vi "VG_Array_OCVCELL.vi"() -> ()   [LabVIEW 2020]
panel:
  out "OCV Cells":dbl[](array[numeric])
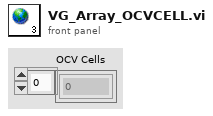
[diagram p1: front panel]
diagram:
